vi "Header Footer Create Cell.vi"(0 "Change format?":bool, 1 "Header or Footer":T10, 2 "FixedHeight (points)":sgl, 3 "Padding (points)":sgl, 7 "Header Footer Cluster with references IN":T1={"Start page"=1, "Type"=enum."Select", "Alignment"=enum."Center", "Vertical Alignement"=enum."MIDDLE", "Page #"={"Text 1"="", "Text 2"="", "Text 3"=""}, "Text"=refnum, "Scaled Img"=refnum, "PdfPCell"=refnum, "PdfPTable"=refnum, "Font Cluster"={"Name"="", "Size"=-1.0, "Color"=0, "Style"={"Bold"=FALSE, "Italic"=FALSE, "Underline"=FALSE, "Strikeout"=FALSE}}, "Font "=refnum, "Img (%)"=100.0, "Line"={"Line"=enum."Horizontal line", "Thickness (points)"=0.75, "Colour"=7171459}}, 11 "error in (no error)":errorcluster) -> (4 "PdfP Cell":refnum<k24>, 8 "Header Footer Cluster with references OUT":T1={"Start page"=1, "Type"=enum."Select", "Alignment"=enum."Center", "Vertical Alignement"=enum."MIDDLE", "Page #"={"Text 1"="", "Text 2"="", "Text 3"=""}, "Text"=refnum, "Scaled Img"=refnum, "PdfPCell"=refnum, "PdfPTable"=refnum, "Font Cluster"={"Name"="", "Size"=-1.0, "Color"=0, "Style"={"Bold"=FALSE, "Italic"=FALSE, "Underline"=FALSE, "Strikeout"=FALSE}}, "Font "=refnum, "Img (%)"=100.0, "Line"={"Line"=enum."Horizontal line", "Thickness (points)"=0.75, "Colour"=7171459}}, 15 "error out":errorcluster)   [LabVIEW 2013]
doc: "Version 1.0\nDeveloped by Jean-Marc Simard\nCopyright © 2010, Exaprom Inc.\nAll rights reserved.\nLicense: BSD\n\nWith iTextSharp 4.1.6 (http://itextsharp.sourceforge.net)\nunder Mozilla Public License Version 1.1\n(http://www.mozilla.org/MPL/MPL-1.1.html)"
uses:
  C:/Users/MaxCorp/Documents/GitHub/TopView/DLL/itextsharp.dll
  DLL/itextsharp.dll
  Controls/Header Footer Cluster with references.ctl
  Controls/Header Footer Type.ctl
  Controls/Header footer horiz alignment.ctl
  Controls/Cell Vertical alignment.ctl
  Controls/Page number.ctl
  Controls/Font cluster.ctl
  Controls/Font size.ctl
  Controls/Font color.ctl
  Controls/Header Footer Line.ctl
  Controls/Header or Footer.ctl
panel:
  # "X"
  # "Y"
  # "X"
  # "Y"
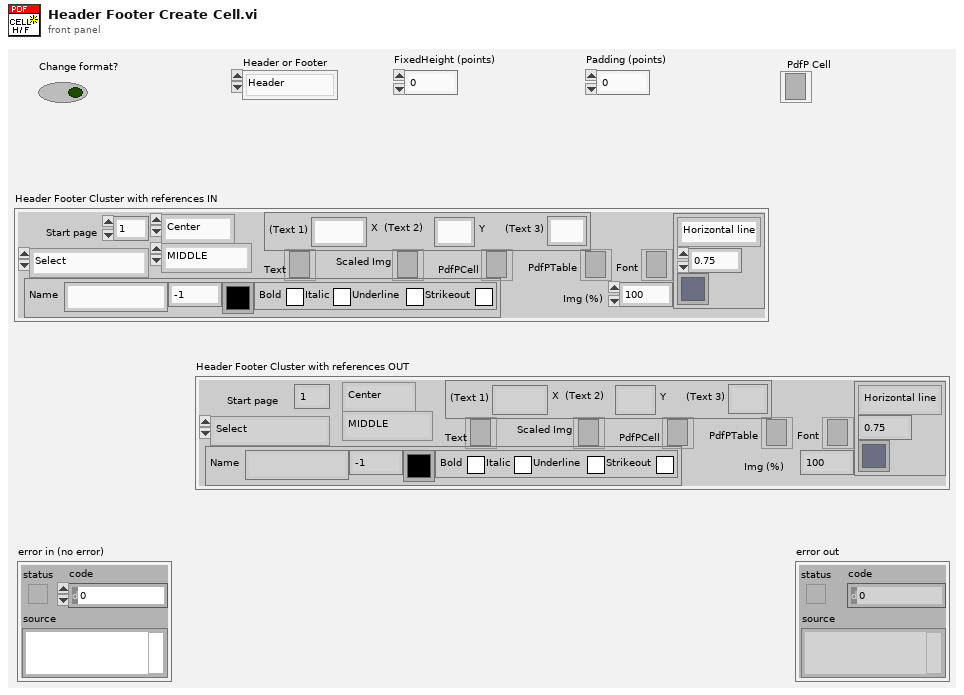
[diagram p1: front panel]
types:
  T1 = typedef "Header Footer Cluster with references.ctl" = cluster{"Start page":i32, "Type":T2, "Alignment":T3, "Vertical Alignement":T4, "Page #":T5, "Text":refnum<k24>, "Scaled Img":refnum<k24>, "PdfPCell":refnum<k24>, "PdfPTable":refnum<k24>, "Font Cluster":T6, "Font ":refnum<k24>, "Img (%)":sgl, "Line":cluster{"Line":T9, "Thickness (points)":sgl, "Colour":T8}}
  T2 = typedef "Header Footer Type.ctl" = enum16{"Select", "Text", "Text + hyperlink", "Page number", "Image", "Image + hyperlink"}
  T3 = typedef "Header footer horiz alignment.ctl" = enum16{"Left", "Center", "Right"}
  T4 = typedef "Cell Vertical alignment.ctl" = enum16{"TOP", "MIDDLE", "BOTTOM"}
  T5 = typedef "Page number.ctl" = cluster{"Text 1":string, "Text 2":string, "Text 3":string}
  T6 = typedef "Font cluster.ctl" = cluster{"Name":string, "Size":T7, "Color":T8, "Style":cluster{"Bold":bool, "Italic":bool, "Underline":bool, "Strikeout":bool}}
  T7 = typedef "Font size.ctl" = sgl
  T8 = typedef "Font color.ctl" = u32
  T9 = typedef "Header Footer Line.ctl" = enum16{"No line", "Horizontal line"}
  T10 = typedef "Header or Footer.ctl" = enum16{"Header", "Footer"}
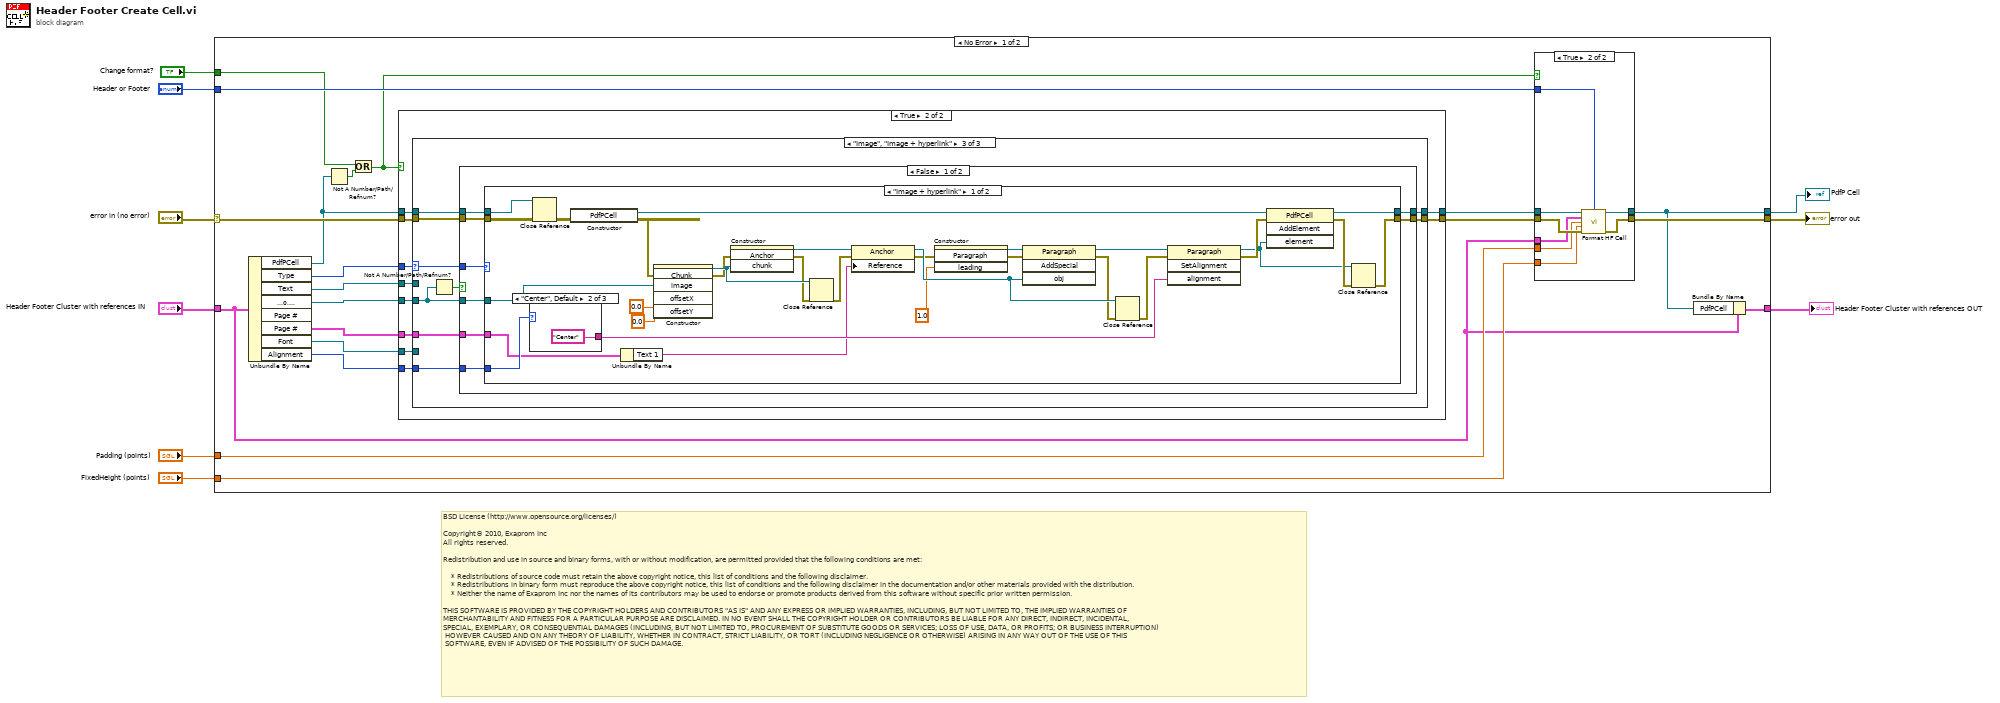
[diagram p0: block diagram]
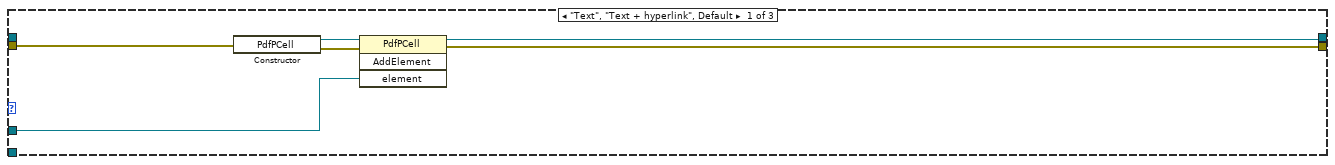
[diagram p3: hidden frame]
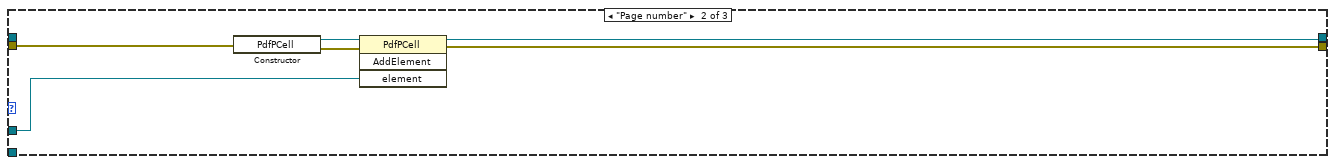
[diagram p4: hidden frame]
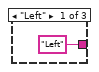
[diagram p5: hidden frame]
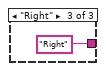
[diagram p6: hidden frame]
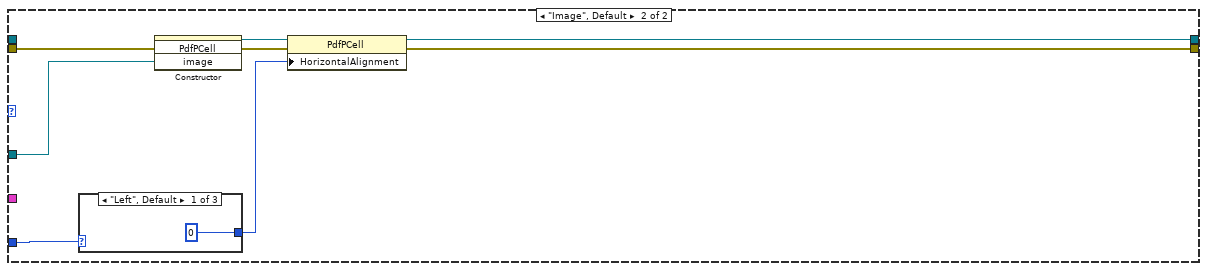
[diagram p7: hidden frame]
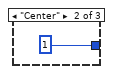
[diagram p8: hidden frame]
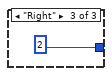
[diagram p9: hidden frame]
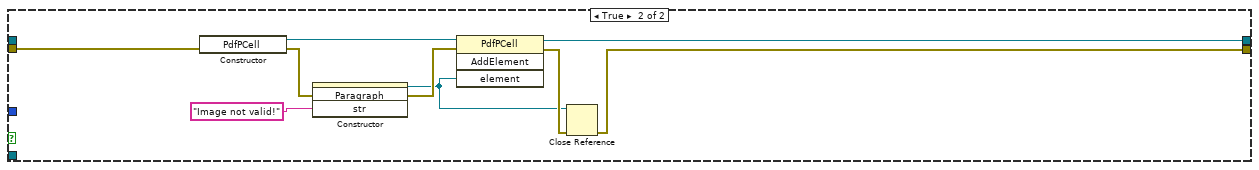
[diagram p10: hidden frame]
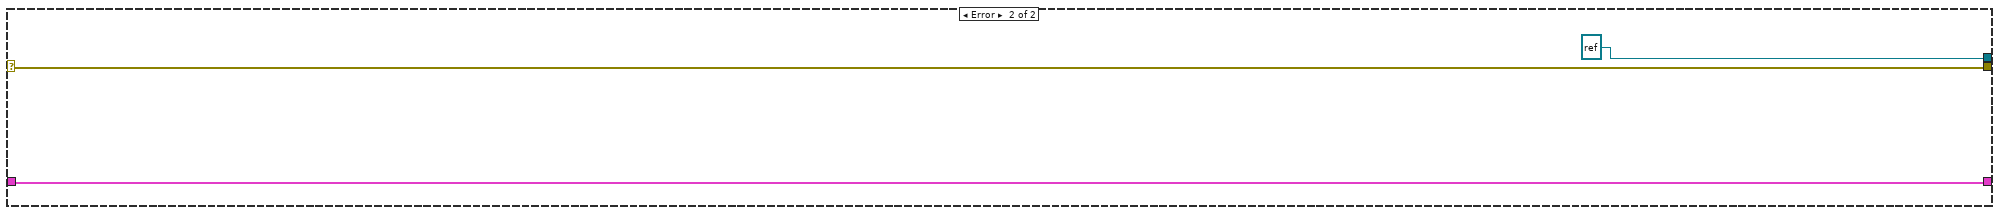
[diagram p12: hidden frame]
diagram:
  # "BSD License (http://www.opensource.org/licenses/)\n\nCopyright© 2010, Exaprom Inc\nAll rights reserved.\n\nRedistribution and use in source and binary forms, with or without modification, are permitted provided that the following conditions are met:\n\n    * Redistributions of source code must retain the above copyright notice, this list of conditions and the following disclaimer.\n    * Redistributions in binary form must reproduce the above copyright notice, this list of conditions and the following disclaimer in the documentation and/or other materials provided with the distribution.\n    * Neither the name of Exaprom Inc nor the names of its contributors may be used to endorse or promote products derived from this software without specific prior written permission.\n\nTHIS SOFTWARE IS PROVIDED BY THE COPYRIGHT HOLDERS AND CONTRIBUTORS \"AS IS\" AND ANY EXPRESS OR IMPLIED WARRANTIES, INCLUDING, BUT NOT LIMITED TO, THE IMPLIED WARRANTIES OF \nMERCHANTABILITY AND FITNESS FOR A PARTICULAR PURPOSE ARE DISCLAIMED. IN NO EVENT SHALL THE COPYRIGHT HOLDER OR CONTRIBUTORS BE LIABLE FOR ANY DIRECT, INDIRECT, INCIDENTAL,\nSPECIAL, EXEMPLARY, OR CONSEQUENTIAL DAMAGES (INCLUDING, BUT NOT LIMITED TO, PROCUREMENT OF SUBSTITUTE GOODS OR SERVICES; LOSS OF USE, DATA, OR PROFITS; OR BUSINESS INTERRUPTION)\n HOWEVER CAUSED AND ON ANY THEORY OF LIABILITY, WHETHER IN CONTRACT, STRICT LIABILITY, OR TORT (INCLUDING NEGLIGENCE OR OTHERWISE) ARISING IN ANY WAY OUT OF THE USE OF THIS\n SOFTWARE, EVEN IF ADVISED OF THE POSSIBILITY OF SUCH DAMAGE."
  n1 = case shown="No Error" "error in (no error)" {
    selector: "error in (no error)" -> [w29 w136]
    tunnel: [w12 refnum<k24> refnum ("new reference")] -> w9
    tunnel: [w22 w136] -> w8
    tunnel: "Header Footer Cluster with references IN" -> [w13 w134]
    tunnel: "Padding (points)" -> [w21 _]
    tunnel: "FixedHeight (points)" -> [w20 _]
    tunnel: "Header or Footer" -> [w19 _]
    tunnel: "Change format?" -> [w11 _]
    tunnel: [w14 w134] -> w1
    frame No Error {
      n2 = Unbundle By Name(w13) -> ("PdfPCell"=w17:refnum<k24>, "Type"=w16:T2, "Text"=w27:refnum<k24>, "Scaled Img"=w28:refnum<k24>, "Page #"=w18:T5, "Font"=w26:refnum<k24>, "Alignment"=w25:T3)  [unwired: 1 out]
      n3 = Not A Number/Path/Refnum?(number/path/refnum=w17) -> (NaN/Path/Refnum?=w15:bool)
      n4 = Or(x=w11, y=w15) -> (x .or. y?=w10:bool)
      n5 = case shown="True" w10 {
        tunnel: [w31 w41] -> w24
        tunnel: [w30 w40] -> w23
        tunnel: w16 -> [_ w39]
        tunnel: w29 -> [w30 w38]
        tunnel: w28 -> [_ w37]
        tunnel: w18 -> [_ w36]
        tunnel: w27 -> [_ w35]
        tunnel: w26 -> [_ w34]
        tunnel: w25 -> [_ w33]
        tunnel: w17 -> [w31 w32]
        frame False {
        }
        frame True {
          n6 = case shown="\"Image\", \"Image + hyperlink\"" w39 {
            selector: w39 -> [_ _ w59]
            tunnel: [w45 w52 w62] -> w41
            tunnel: w34 -> [_ _ _]
            tunnel: w33 -> [_ _ w60]
            tunnel: [w44 w51 w61] -> w40
            tunnel: w38 -> [w46 w53 w58]
            tunnel: w37 -> [_ _ w56]
            tunnel: w36 -> [_ _ w57]
            tunnel: w35 -> [w47 w48 _]
            tunnel: w32 -> [_ _ w54]
            frame "Text", "Text + hyperlink", Default {
              n7 = constructor class="PdfPCell"(error in=w46) -> (reference out=w42:refnum<k24>, error out=w43:errorcluster)  [unwired: 2 in, 1 out]
              n8 = invoke class="PdfPCell" method="AddElement"(reference=w42, error in=w43, "element"=w47) -> (reference out=w45:refnum<k24>, error out=w44:errorcluster)  [unwired: 1 in, 2 out]
            }
            frame "Page number" {
              n9 = constructor class="PdfPCell"(error in=w53) -> (reference out=w49:refnum<k24>, error out=w50:errorcluster)  [unwired: 2 in, 1 out]
              n10 = invoke class="PdfPCell" method="AddElement"(reference=w49, error in=w50, "element"=w48) -> (reference out=w52:refnum<k24>, error out=w51:errorcluster)  [unwired: 1 in, 2 out]
            }
            frame "Image", "Image + hyperlink" {
              n11 = Not A Number/Path/Refnum?(number/path/refnum=w56) -> (NaN/Path/Refnum?=w55:bool)
              n12 = case shown="False" w55 {
                tunnel: [w68 w116] -> w61
                tunnel: [w69 w120] -> w62
                tunnel: w60 -> [w70 _]
                tunnel: w59 -> [w67 _]
                tunnel: w58 -> [w65 w115]
                tunnel: w56 -> [w66 _]
                tunnel: w57 -> [w64 _]
                tunnel: w54 -> [w63 _]
                frame False {
                  n13 = case shown="\"Image + hyperlink\"" w67 {
                    tunnel: w70 -> [w78 w111]
                    tunnel: [w80 w108] -> w69
                    tunnel: w65 -> [w79 w106]
                    tunnel: [w77 w104] -> w68
                    tunnel: w64 -> [w76 _]
                    tunnel: w66 -> [w74 w105]
                    tunnel: w63 -> [w71 _]
                    frame "Image + hyperlink" {
                      n14 = case shown="\"Center\", Default" w78 {
                        tunnel: ["Left" "Center" "Right"] -> w97
                        frame "Left" {
                        }
                        frame "Center", Default {
                        }
                        frame "Right" {
                        }
                      }
                      n15 = Close Reference(reference=w71, error in (no error)=w79) -> (error out=w72:errorcluster)
                      n16 = constructor class="PdfPCell"(error in=w72) -> (reference out=w96:refnum<k24>, error out=w85:errorcluster)  [unwired: 2 in, 1 out]
                      n17 = Unbundle By Name(w76) -> ("Text 1"=w73:string)
                      n18 = constructor class="Chunk"(error in=w85, "image"=w74, "offsetX"=sgl 0.0, "offsetY"=sgl 0.0) -> (reference out=w100:refnum<k24>, error out=w81:errorcluster)  [unwired: 2 in, 4 out]
                      n19 = constructor class="Anchor"(error in=w81, "chunk"=w100) -> (reference out=w84:refnum<k24>, error out=w98:errorcluster)  [unwired: 2 in, 2 out]
                      n20 = Close Reference(reference=w100, error in (no error)=w98) -> (error out=w99:errorcluster)
                      n21 = property class="Anchor"(reference=w84, error in=w99, "Reference"=w73) -> (reference out=w95:refnum<k24>, error out=w94:errorcluster)
                      n22 = constructor class="Paragraph"(error in=w94, "leading"=sgl 1.0) -> (reference out=w90:refnum<k24>, error out=w91:errorcluster)  [unwired: 2 in, 2 out]
                      n23 = invoke class="Paragraph" method="AddSpecial"(reference=w90, error in=w91, "obj"=w95) -> (reference out=w92:refnum<k24>, error out=w89:errorcluster)  [unwired: 1 in, 2 out]
                      n24 = Close Reference(reference=w95, error in (no error)=w89) -> (error out=w88:errorcluster)
                      n25 = invoke class="Paragraph" method="SetAlignment"(reference=w92, error in=w88, "alignment"=w97) -> (reference out=w86:refnum<k24>, error out=w93:errorcluster)  [unwired: 1 in, 2 out]
                      n26 = invoke class="PdfPCell" method="AddElement"(reference=w96, error in=w93, "element"=w86) -> (reference out=w80:refnum<k24>, error out=w87:errorcluster)  [unwired: 1 in, 2 out]
                      n27 = Close Reference(reference=w86, error in (no error)=w87) -> (error out=w77:errorcluster)
                    }
                    frame "Image", Default {
                      n28 = case shown="\"Left\", Default" w111 {
                        tunnel: [0 1 2] -> w107
                        frame "Left", Default {
                        }
                        frame "Center" {
                        }
                        frame "Right" {
                        }
                      }
                      n29 = constructor class="PdfPCell"(error in=w106, "image"=w105) -> (reference out=w110:refnum<k24>, error out=w109:errorcluster)  [unwired: 2 in, 2 out]
                      n30 = property class="PdfPCell"(reference=w110, error in=w109, "HorizontalAlignment"=w107) -> (reference out=w108:refnum<k24>, error out=w104:errorcluster)
                    }
                  }
                }
                frame True {
                  n31 = constructor class="PdfPCell"(error in=w115) -> (reference out=w121:refnum<k24>, error out=w123:errorcluster)  [unwired: 2 in, 1 out]
                  n32 = constructor class="Paragraph"(error in=w123, "str"="Image not valid!") -> (reference out=w117:refnum<k24>, error out=w122:errorcluster)  [unwired: 2 in, 2 out]
                  n33 = invoke class="PdfPCell" method="AddElement"(reference=w121, error in=w122, "element"=w117) -> (reference out=w120:refnum<k24>, error out=w118:errorcluster)  [unwired: 1 in, 2 out]
                  n34 = Close Reference(reference=w117, error in (no error)=w118) -> (error out=w116:errorcluster)
                }
              }
            }
          }
        }
      }
      n35 = case shown="True" w10 {
        tunnel: w24 -> [w125 w133]
        tunnel: w23 -> [w124 w131]
        tunnel: [w125 w132] -> w12
        tunnel: [w124 w130] -> w22
        tunnel: w13 -> [_ w129]
        tunnel: w21 -> [_ w128]
        tunnel: w20 -> [_ w127]
        tunnel: w19 -> [_ w126]
        frame False {
        }
        frame True {
          n36 = call "Format HF Cell.vi"("PdfP Cell"=w133, "Header or Footer"=w126, "Header Footer Cluster with references"=w129, "Padding (points)"=w128, "FixedHeight (points)"=w127, "error in (no error)"=w131) -> ("PdfP Cell duplicate"=w132:refnum<k24>, "error out"=w130:errorcluster)  [unwired: 8 out]
        }
      }
      n37 = Bundle By Name(cluster=w13, "PdfPCell"=w12) -> (w14:T1)
    }
    frame Error {
    }
  }
  "PdfP Cell" <- w9
  "error out" <- w8
  "Header Footer Cluster with references OUT" <- w1
